vi "Full Data Write Subroutine.vi"() -> ()   [LabVIEW 2020]
uses:
  Data Handling Operations/Data Clusters/Database Information.ctl
  Data Handling Operations/Data Clusters/Layer Information Cluster.ctl
  <vilib>/addons/database/Connection.llb/Conn ObjectReference.ctl
  <vilib>/addons/database/NI_Database_API.lvlib
panel:
  in  "Database Full Information In":T1 {"Database Write Information"."Layer Information Array"."Deposition Method" items=["Blade Coating", "Spin Coating", "Thermal Evaporation", "E-Beam Evaporation", "Sputtering", "Drop Casting", "Dip Coating", "Pulsed Laser Deposition", "Chemival Vapour Deposition", "Atomic Layer Deposition", "Spray Coating", "Screen Printing", "Electroplating", "Molecular Beam Epitaxy", "Custom Deposition"]; "Database Write Information"."Layer Information Array"."Layer Type" items=["Front Electrode", "Electron Transport Layer", "Active Layer", "Hole Transport Layer", "Back Electrode", "Custom Layer"]}
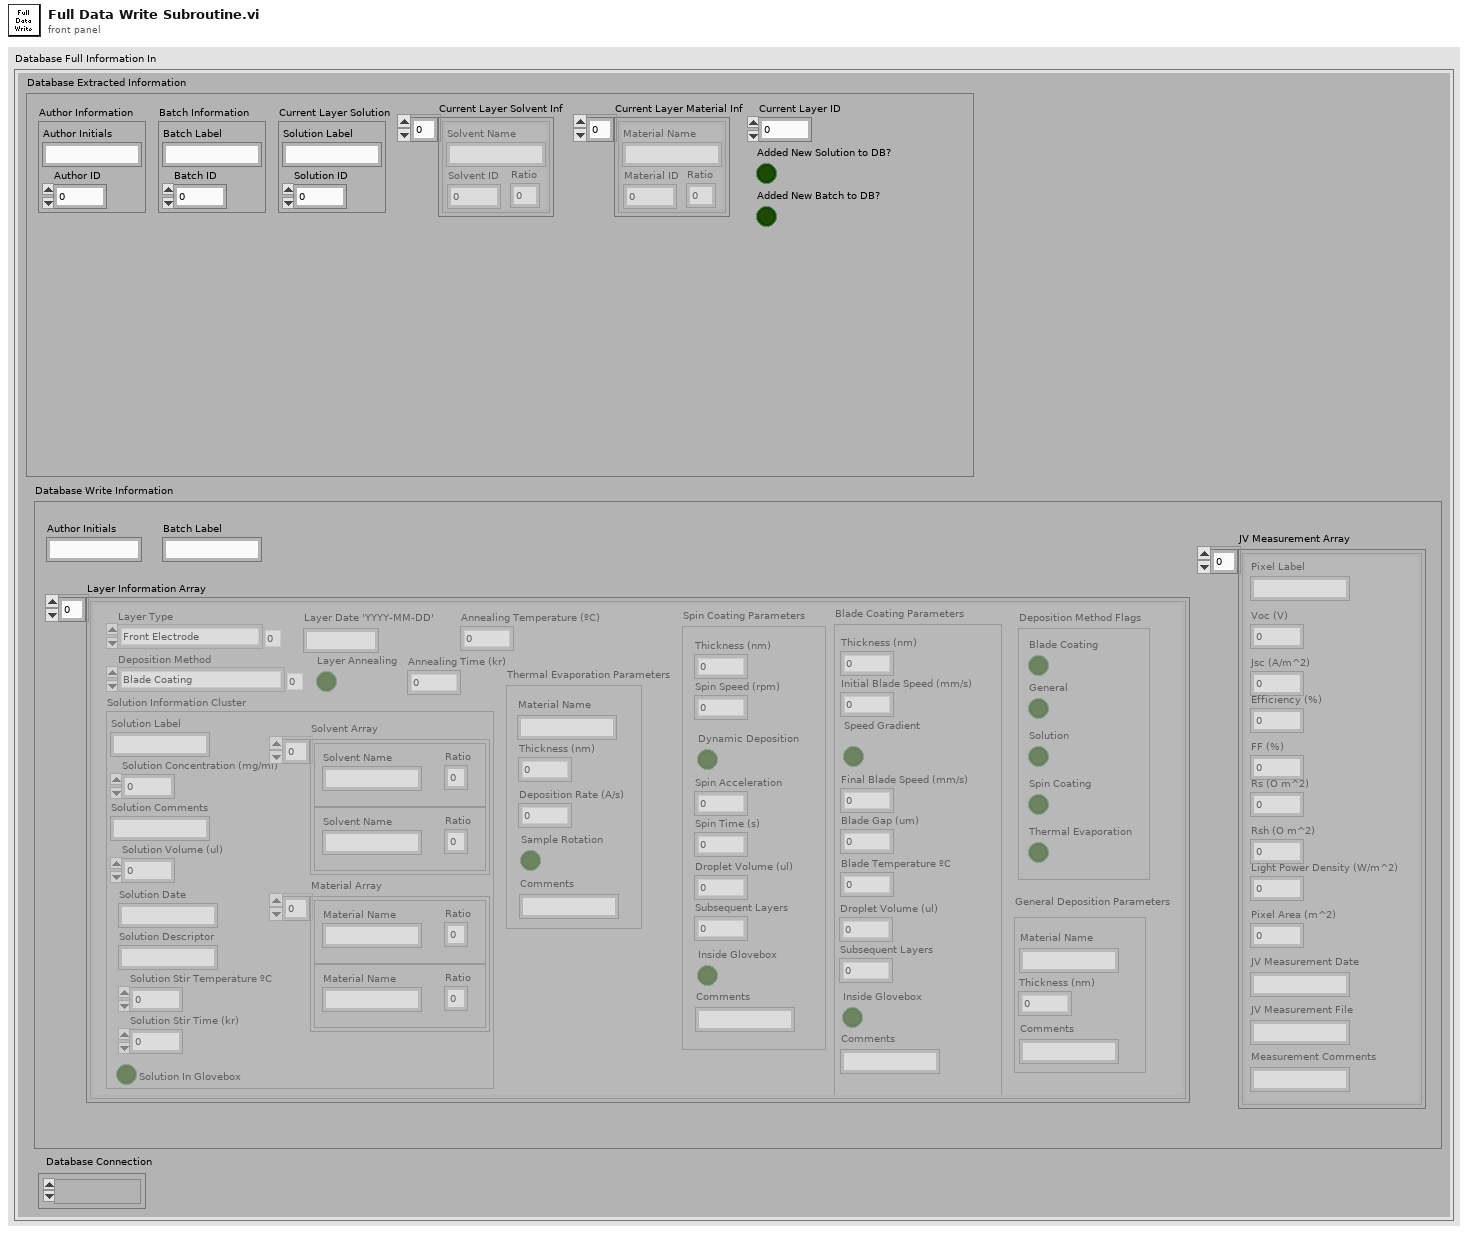
[diagram p1: front panel]
types:
  T1 = typedef "Database Information.ctl" = cluster{"Database Extracted Information":cluster{"Author Information":cluster{"Author Initials":string, "Author ID":i32}, "Batch Information":cluster{"Batch Label":string, "Batch ID":i32}, "Current Layer Solution":cluster{"Solution Label":string, "Solution ID":i32}, "Current Layer ID":i32, "Current Layer Solvent Inf":cluster{"Solvent Name":string, "Solvent ID":i32, "Ratio":dbl}[], "Current Layer Material Inf":cluster{"Material Name":string, "Material ID":i32, "Ratio":dbl}[], "Added New Solution to DB?":bool, "Added New Batch to DB?":bool}, "Database Write Information":cluster{"Author Initials":string, "Batch Label":string, "Layer Information Array":T2[], "JV Measurement Array":cluster{"Pixel Label":string, "Voc (V) ":dbl, "Jsc (A/m^2) ":dbl, "Efficiency (%)":dbl, "FF (%)":dbl, "Rs (O m^2)":dbl, "Rsh (O m^2)":dbl, "Light Power Density (W/m^2)":dbl, "Pixel Area (m^2)":dbl, "JV Measurement Date":string, "JV Measurement File":string, "Measurement Comments":string}[]}, "Database Connection":T3}
  T2 = typedef "Layer Information Cluster.ctl" = cluster{"Solution Information Cluster":cluster{"Solution Label":string, "Solution Concentration (mg/ml)":dbl, "Solution Comments ":string, "Solution Volume (ul) ":dbl, "Solution Date ":string, "Solution Descriptor ":string, "Solution Stir Temperature ºC ":dbl, "Solution Stir Time (kr) ":dbl, "Solution In Glovebox":bool, "Solvent Array":cluster{"Solvent Name":string, "Ratio":dbl}[], "Material Array":cluster{"Material Name":string, "Ratio":dbl}[]}, "Layer Type":u16, "Deposition Method":u16, "Layer Annealing":bool, "General Deposition Parameters":cluster{"Thickness (nm)":dbl, "Comments":string, "Material Name":string}, "Blade Coating Parameters":cluster{"Thickness (nm)":dbl, "Initial Blade Speed (mm/s)":dbl, "Speed Gradient":bool, "Final Blade Speed (mm/s)":dbl, "Blade Gap (um)":dbl, "Droplet Volume (ul)":dbl, "Subsequent Layers":dbl, "Inside Glovebox":bool, "Comments":string, "Blade Temperature ºC":dbl}, "Spin Coating Parameters":cluster{"Thickness (nm)":dbl, "Spin Speed (rpm)":dbl, "Dynamic Deposition":bool, "Spin Acceleration":dbl, "Spin Time (s)":dbl, "Droplet Volume (ul)":dbl, "Subsequent Layers":dbl, "Inside Glovebox":bool, "Comments":string}, "Thermal Evaporation Parameters":cluster{"Deposition Rate (A/s)":dbl, "Thickness (nm)":dbl, "Comments":string, "Material Name":string, "Sample Rotation":bool}, "Layer Date 'YYYY-MM-DD'":string, "Annealing Time (kr)":dbl, "Annealing Temperature (ºC)":dbl, "Deposition Method Flags":cluster{"Blade Coating":bool, "General ":bool, "Solution":bool, "Spin Coating":bool, "Thermal Evaporation":bool}}
  T3 = typedef "NI_Database_API.lvlib/Conn ObjectReference.ctl" = refnum<k1>
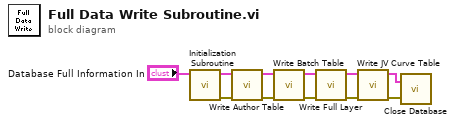
[diagram p0: block diagram]
diagram:
  n1 = call "Initialization Subroutine.vi"("Database Full Information In"="Database Full Information In") -> ("Error Out"=w10:errorcluster, "Database Full Information Out"=w9:T1)  [unwired: 9 in]
  n2 = call "Write Author Table.vi"("Error In"=w10, "Database Full Information In"=w9) -> ("Error Out"=w8:errorcluster, "Database Full Information Out"=w7:T1)  [unwired: 8 in]
  n3 = call "Write Batch Table.vi"("Error In"=w8, "Database Full Information In"=w7) -> ("Error Out"=w6:errorcluster, "Database Full Information Out"=w5:T1)  [unwired: 8 in]
  n4 = call "Write Full Layer.vi"("Error In"=w6, "Database Full Information In"=w5) -> ("Error Out"=w3:errorcluster, "Database Full Information Out"=w4:T1)  [unwired: 8 in]
  n5 = call "Write JV Curve Table.vi"("Error In"=w3, "Database Full Information In"=w4) -> ("Error Out"=w2:errorcluster, "Database Full Information Out"=w1:T1)  [unwired: 8 in]
  n6 = call "Close Database.vi"("Error In"=w2, "Database Full Information In"=w1) -> ()  [unwired: 1 in, 1 out]
